vi "Set Control Value by Name.vi"(8 "错误输入（无错误）":errorcluster, 9 "Value":variant, 10 "Control Name":string, 11 "VI Ref":refnum<vi>) -> (0 "错误输出":errorcluster)   [LabVIEW 2012, in "VIRef.lvlib"]
uses:
  VIRef.lvlib
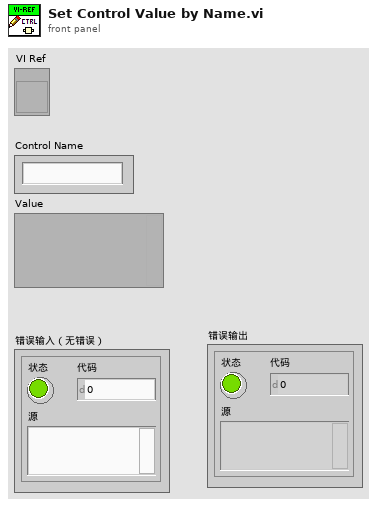
[diagram p1: front panel]
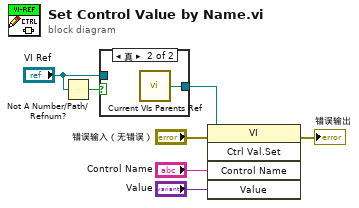
[diagram p0: block diagram]
diagram:
  n1 = Not A Number/Path/Refnum?(number/path/refnum="VI Ref") -> (NaN/Path/Refnum?=w6:bool)
  n2 = case shown="真" w6 {
    tunnel: [w8 w9] -> w5
    tunnel: "VI Ref" -> [w8 _]
    frame False {
    }
    frame True {
      n3 = call "Current VIs Parents Ref.vi"() -> ("Calling VI's Reference"=w9:refnum<vi>)  [unwired: 2 in]
    }
  }
  n4 = invoke class="VI" method="Ctrl Val.Set"(reference=w5, error in="错误输入（无错误）", "Control Name"="Control Name", "Value"="Value") -> (error out=→"错误输出":errorcluster)  [unwired: 1 in, 4 out]
